vi "KE622x -- Get Buffer Stats Params.vi"(0 "Resource In":refnum<visa-resource-name>, 1 "Check For SCPI Errors? (T)":bool=TRUE, 11 "error in (no error)":errorcluster) -> (4 "Resource Out (dupl)":refnum<visa-resource-name>, 8 "Buffer Stats Params":T1={"Stats Enabled?"=FALSE, "Stats Mode"=enum."Std Dev"}, 15 "error out":errorcluster)   [LabVIEW 2019, in "Keithley 622x.lvlib"]
doc: "Returns the type of buffer statistics calculation the instrument will perform on readings stored in the trace buffer (Mean, Standard Deviation, Min, Max, or Peak-to-Peak), and also whether or not the statistics calculation is enabled."
uses:
  Keithley 622x.lvlib
  Typedefs/KE622x -- Buffer Stats Params.ctl
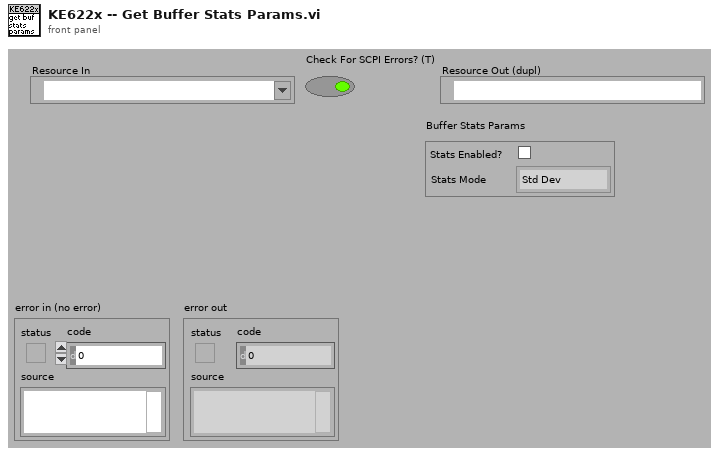
[diagram p1: front panel]
types:
  T1 = typedef "Keithley 622x.lvlib/KE622x -- Buffer Stats Params.ctl" = cluster{"Stats Enabled?":bool, "Stats Mode":enum16{"Mean", "Std Dev", "Max", "Min", "Peak-to-Peak"}}
  T2 = enum16{"Mean", "Std Dev", "Max", "Min", "Peak-to-Peak"}
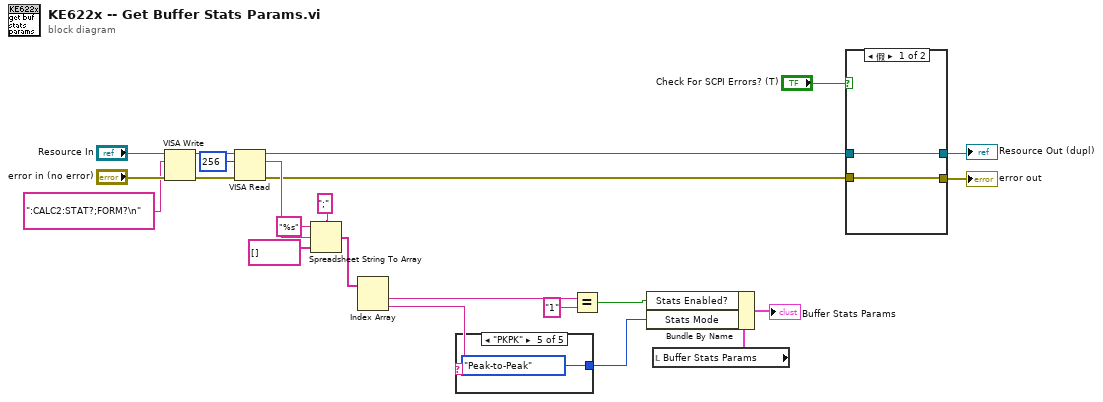
[diagram p0: block diagram]
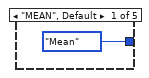
[diagram p2: hidden frame]
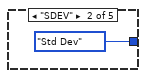
[diagram p3: hidden frame]
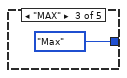
[diagram p4: hidden frame]
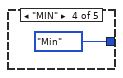
[diagram p5: hidden frame]
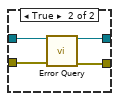
[diagram p6: hidden frame]
diagram:
  n1 = VISA Write(VISA resource name="Resource In", write buffer=":CALC2:STAT?;FORM?\n" ("format string"), error in (no error)="error in (no error)") -> (VISA resource name out=w17:refnum<visa-resource-name>, error out=w16:errorcluster)  [unwired: 1 out]
  n2 = VISA Read(VISA resource name=w17, byte count=u32 256, error in (no error)=w16) -> (VISA resource name out=w14:refnum<visa-resource-name>, read buffer=w13:string, error out=w2:errorcluster)  [unwired: 1 out]
  n3 = Spreadsheet String To Array(delimiter (Tab)=";", format string="%s", spreadsheet string=w13, array type (2D Dbl)=string[] []) -> (array=w9:string[])
  n4 = Index Array(array=w9) -> (element #1=w8:string, element #2=w3:string)  [unwired: 2 in]
  n5 = case shown="\"PKPK\"" w3 {
    tunnel: [T2."Mean" ("Stats Mode") T2."Std Dev" ("Stats Mode") T2."Max" ("Stats Mode") T2."Min" ("Stats Mode") T2."Peak-to-Peak" ("Stats Mode")] -> w1
    frame "MEAN", Default {
    }
    frame "SDEV" {
    }
    frame "MAX" {
    }
    frame "MIN" {
    }
    frame "PKPK" {
    }
  }
  n6 = Equal?(x=w8, y="1") -> (x = y?=w5:bool)
  n7 = local read "Buffer Stats Params"() -> (w6:T1)
  n8 = Bundle By Name(cluster=w6, "Stats Enabled?"=w5, "Stats Mode"=w1) -> (→"Buffer Stats Params":T1)
  n9 = case shown="假" "Check For SCPI Errors? (T)" {
    tunnel: w14 -> [w30 w34]
    tunnel: w2 -> [w29 w33]
    tunnel: [w29 w32] -> w19
    tunnel: [w30 w31] -> w20
    frame False {
    }
    frame True {
      n10 = call "Error Query.vi"("VISA Resource In"=w34, "error in (no error)"=w33) -> ("VISA Resource Out (dupl)"=w31:refnum<visa-resource-name>, "error out"=w32:errorcluster)  [unwired: 10 in, 2 out]
    }
  }
  "Resource Out (dupl)" <- w20
  "error out" <- w19
